vi "DHE_ReadTPs.vi"(5 "inRange":bool, 6 "index in":i32, 7 "value":string, 8 "error in (no error)":errorcluster, 9 "argument":string, 10 "action":T3=enum."GET ALL", 11 "file path":path=path "/home/arcconfig/TP_DHE.list") -> (0 "error out":errorcluster, 1 "index":i32[](array[numeric]), 2 "TPs":T1[](array[typedef]) {"Limits"."nominal" format="%.2f"; "Limits"."Lower" format="%.2f"; "Limits"."upper" format="%.2f"}, 3 "file path out":path=path "/home/ArcVIEW/ConfigFiles/PI_laboratory.cfg", 4 "devparams":string)   [LabVIEW 2016]
uses:
  DHE_TP_action.ctl
  DHE_TP.ctl
  DHE_TPLimits.ctl
  <vilib>/Utility/config.llb/Read Key (String).vi
  <vilib>/Utility/config.llb/NI_LVConfig.lvlib
panel:
  in  "DHE_TP":T1={"name"="", "type"="", "R_algor"=[], "board"="", "memory"="", "address"=0, "value"="", "Limits"={"upper"=9999999.0, "Lower"=-9999999.0, "InRange"=FALSE, "nominal"=0.0}, "unit"="", "params"="", "permissions"="RW", "W_algor"=[], "description"="", "err_count"=0, "max_err"=10, "read"=FALSE, "lowrej"=-9999999.0, "hirej"=9999999.0, "expupd"=FALSE} {"Limits"."nominal" format="%.2f"; "Limits"."Lower" format="%.2f"; "Limits"."upper" format="%.2f"}
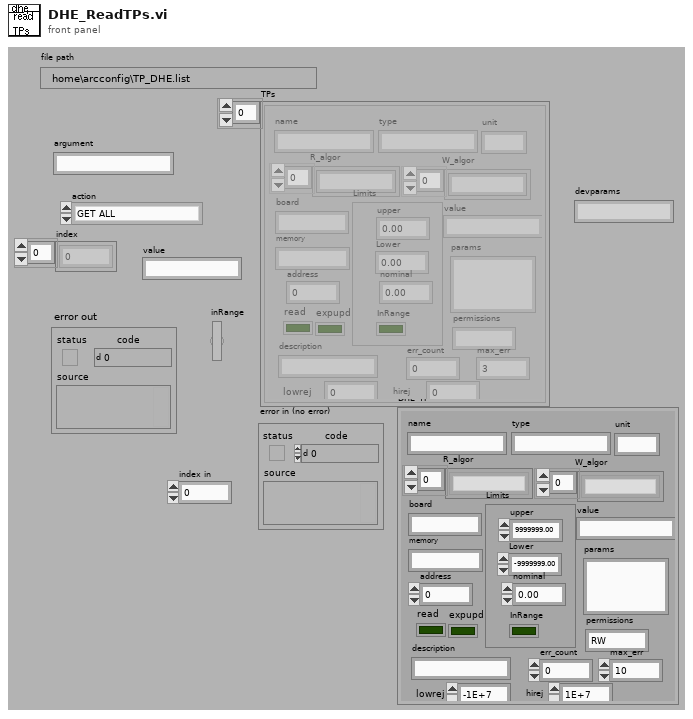
[diagram p1: front panel]
types:
  T1 = typedef "DHE_TP.ctl" = cluster{"name":string, "type":string, "R_algor":string[], "board":string, "memory":string, "address":i32, "value":string, "Limits":T2, "unit":string, "params":string, "permissions":string, "W_algor":string[], "description":string, "err_count":i32, "max_err":i32, "read":bool, "lowrej":dbl, "hirej":dbl, "expupd":bool}
  T2 = typedef "DHE_TPLimits.ctl" = cluster{"upper":dbl, "Lower":dbl, "InRange":bool, "nominal":dbl}
  T3 = typedef "DHE_TP_action.ctl" = enum16{"READ FROM FILE", "GET ALL", "FIND BY NAME", "FIND BY TYPE", "SET VALUE", "CLEAN", "CHANGE", "GET EXPUPDATE"}
  T4 = typedef "NI_LVConfig.lvlib/Config Data RefNum.ctl" = refnum<k1>
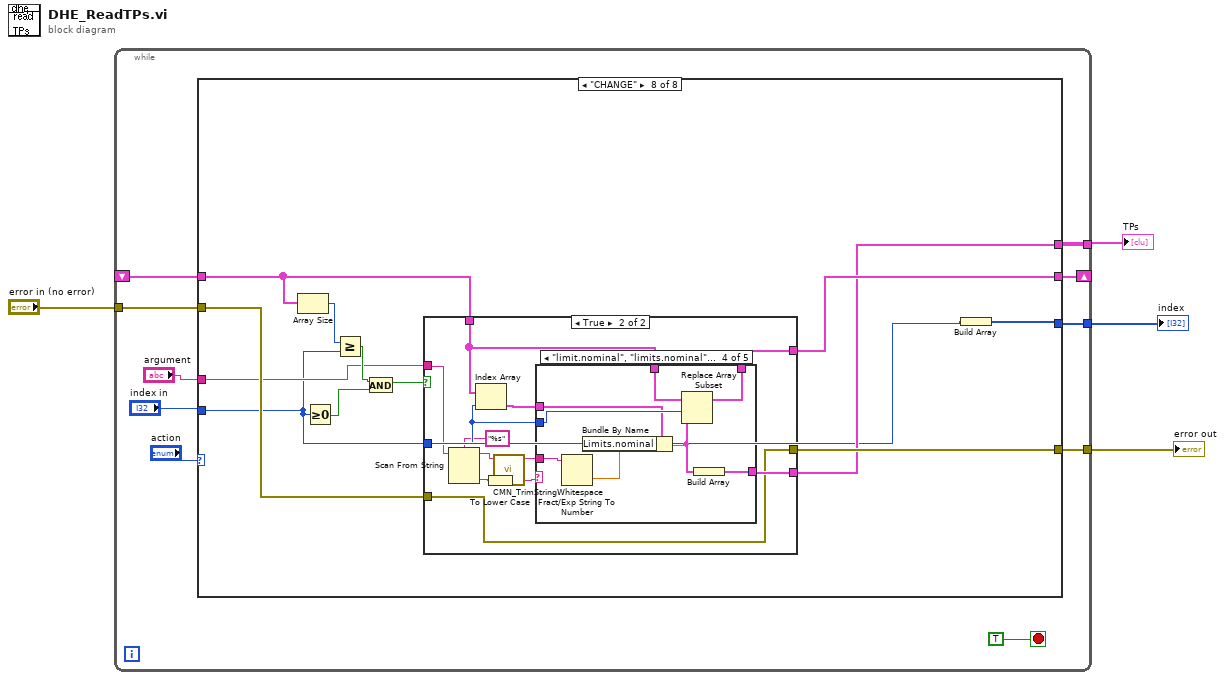
[diagram p0: block diagram]
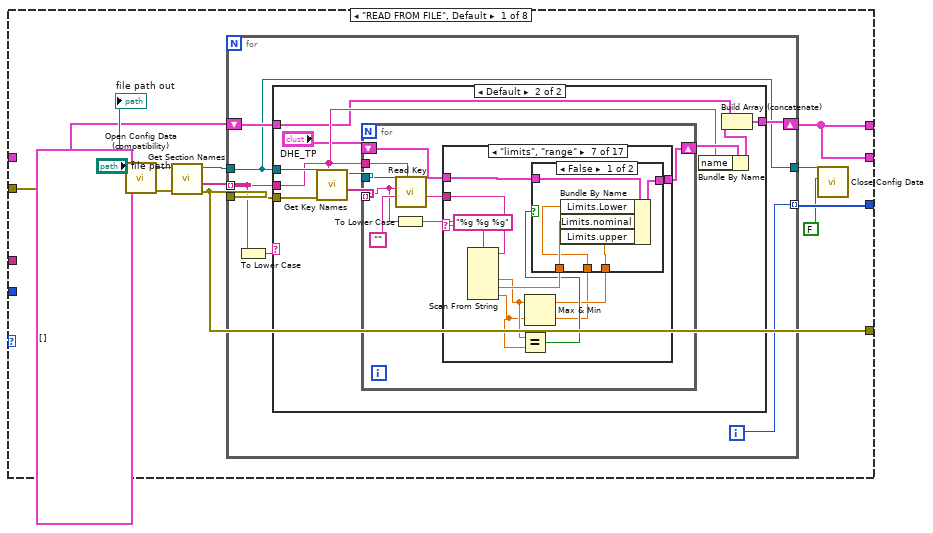
[diagram p2: hidden frame]
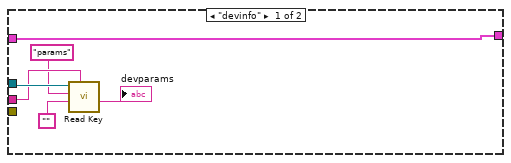
[diagram p3: hidden frame]
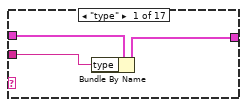
[diagram p4: hidden frame]
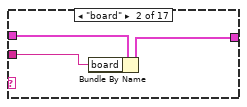
[diagram p5: hidden frame]
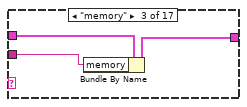
[diagram p6: hidden frame]
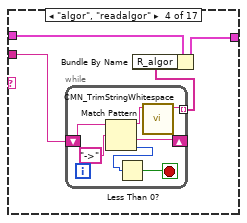
[diagram p7: hidden frame]
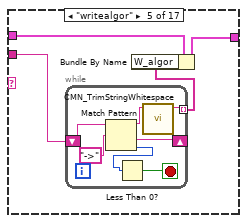
[diagram p8: hidden frame]
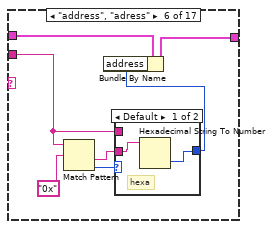
[diagram p9: hidden frame]
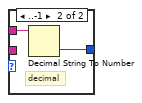
[diagram p10: hidden frame]
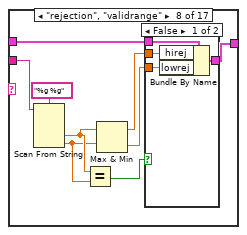
[diagram p12: hidden frame]
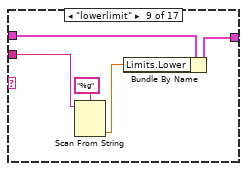
[diagram p14: hidden frame]
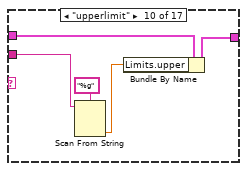
[diagram p15: hidden frame]
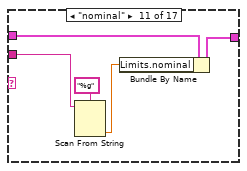
[diagram p16: hidden frame]
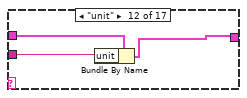
[diagram p17: hidden frame]
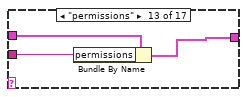
[diagram p18: hidden frame]
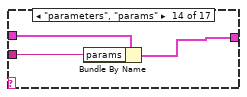
[diagram p19: hidden frame]
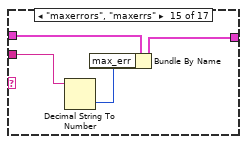
[diagram p20: hidden frame]
diagram:
  n1 = while {
    shift-right: [w11] -> _
    shift-left: _ -> [w10]
    tunnel: "error in (no error)" -> [w12]
    tunnel: [w8] -> w3
    tunnel: [w7] -> w2
    tunnel: [w6] -> w1
    stop <- TRUE stop-if-true
    n2 = case shown="\"CHANGE\"" "action" {
      tunnel: w12 -> [w25 w168 w175 w185 w190 w213 w261 w300]
      tunnel: [w18 w169 w174 w186 w193 w215 w263 w302] -> w11
      tunnel: w10 -> [_ w169 w174 _ w193 w215 w269 w308]
      tunnel: "argument" -> [_ _ _ _ w194 w216 _ w299]
      tunnel: [w20 w166 w170 i32[] [] w187 w211 w259 w297] -> w8
      tunnel: [w18 w169 w172 w186 w191 w214 w262 w301] -> w7
      tunnel: [w19 w168 w175 w185 w189 w212 w264 w303] -> w6
      tunnel: "index in" -> [_ _ _ _ _ _ w260 w298]
      frame "READ FROM FILE", Default {
        n3 = call <vilib>:"Open Config Data (compatibility).vi"("error in (no error)"=w25, "configuration file path"="file path") -> ("error out"=w24:errorcluster, "refnum"=w23:T4)  [unwired: 7 in, 1 out]
        n4 = call <vilib>:"Get Section Names.vi"("error in (no error)"=w24, "refnum"=w23) -> ("error out"=w19:errorcluster, "section names"=w21:string[], "refnum out"=w22:T4)  [unwired: 7 out]
        n5 = for {
          tunnel: w22 -> [w28]
          tunnel: w19 -> [w33]
          tunnel: w21 -> [w32] mode=indexing
          tunnel: [w27] -> w20 mode=indexing
          shift-right: [w30] -> w18
          shift-left: T1[] [] -> [w29]
          tunnel: [w28] -> w16
          i -> [w27]
          n6 = To Lower Case(string=w32) -> (all lower case string=w31:string)
          n7 = case shown="Default" w31 {
            tunnel: w28 -> [w38 w49]
            tunnel: w33 -> [_ w48]
            tunnel: w32 -> [w37 w44]
            tunnel: [w39 w41] -> w30
            tunnel: w29 -> [w39 w40]
            frame "devinfo" {
              n8 = call-poly <vilib>:"Read Key.vi"("section"=w37, "default value"="", "key"="params", "refnum"=w38) -> ("value"=→"devparams":string)  [unwired: 2 in, 5 out]
            }
            frame Default {
              n9 = call <vilib>:"Get Key Names.vi"("section"=w44, "error in (no error)"=w48, "refnum"=w49) -> ("key names"=w47:string[], "refnum out"=w46:T4)  [unwired: 7 out]
              n10 = for {
                tunnel: w47 -> [w53] mode=indexing
                tunnel: w44 -> [w56]
                tunnel: w46 -> [w55]
                shift-right: [w51] -> w45
                shift-left: "DHE_TP" -> [w50]
                n11 = To Lower Case(string=w53) -> (all lower case string=w57:string)
                n12 = call-poly <vilib>:"Read Key.vi"("section"=w56, "default value"="", "key"=w53, "refnum"=w55) -> ("value"=w52:string)  [unwired: 2 in, 5 out]
                n13 = case shown="\"limits\", \"range\"" w57 {
                  tunnel: w50 -> [w60 w63 w66 w70 w81 w95 w109 w119 w134 w139 w144 w147 w150 w153 w157 w162 w165]
                  tunnel: w52 -> [w59 w62 w65 w67 w78 w91 w107 w124 w132 w137 w142 w145 w148 w151 w155 w160 _]
                  tunnel: [w58 w61 w64 w69 w80 w94 w108 w118 w133 w138 w143 w146 w149 w152 w156 w161 w165] -> w51
                  frame "type" {
                    n14 = Bundle By Name(cluster=w60, "type"=w59) -> (w58:T1)
                  }
                  frame "board" {
                    n15 = Bundle By Name(cluster=w63, "board"=w62) -> (w61:T1)
                  }
                  frame "memory" {
                    n16 = Bundle By Name(cluster=w66, "memory"=w65) -> (w64:T1)
                  }
                  frame "algor", "readalgor" {
                    n17 = while {
                      tunnel: [w71] -> w68 mode=indexing
                      shift-right: [w74] -> _
                      shift-left: w67 -> [w73]
                      stop <- w75 stop-if-true
                      n18 = Match Pattern(string=w73, regular expression="->") -> (before substring=w72:string, after substring=w74:string, offset past match=w76:i32)  [unwired: 2 out]
                      n19 = Less Than 0?(x=w76) -> (x < 0?=w75:bool)
                      n20 = call "CMN_TrimStringWhitespace.vi"("string"=w72) -> ("trimmed string"=w71:string)  [unwired: 1 in, 8 out]
                    }
                    n21 = Bundle By Name(cluster=w70, "R_algor"=w68) -> (w69:T1)
                  }
                  frame "writealgor" {
                    n22 = while {
                      tunnel: [w82] -> w79 mode=indexing
                      shift-right: [w85] -> _
                      shift-left: w78 -> [w84]
                      stop <- w86 stop-if-true
                      n23 = Match Pattern(string=w84, regular expression="->") -> (before substring=w83:string, after substring=w85:string, offset past match=w87:i32)  [unwired: 2 out]
                      n24 = Less Than 0?(x=w87) -> (x < 0?=w86:bool)
                      n25 = call "CMN_TrimStringWhitespace.vi"("string"=w83) -> ("trimmed string"=w82:string)  [unwired: 1 in, 8 out]
                    }
                    n26 = Bundle By Name(cluster=w81, "W_algor"=w79) -> (w80:T1)
                  }
                  frame "address", "adress" {
                    n27 = Match Pattern(string=w91, regular expression="0x") -> (after substring=w89:string, offset past match=w92:i32)  [unwired: 3 out]
                    n28 = case shown="Default" w92 {
                      tunnel: w91 -> [_ w99]
                      tunnel: [w96 w98] -> w90
                      tunnel: w89 -> [w97 _]
                      frame Default {
                        # "hexa"
                        n29 = Hexadecimal String To Number(string=w97) -> (number=w96:u32)  [unwired: 3 out]
                      }
                      frame ..-1 {
                        # "decimal"
                        n30 = Decimal String To Number(string=w99) -> (number=w98:i32)  [unwired: 3 out]
                      }
                    }
                    n31 = Bundle By Name(cluster=w95, "address"=w90) -> (w94:T1)
                  }
                  frame "limits", "range" {
                    n32 = Scan From String(format string="%g %g %g", input string=w107) -> (output 1=w104:dbl, output 2=w105:dbl, output 3=w103:dbl)  [unwired: 2 in, 6 out]
                    n33 = Equal?(x=w104, y=w103) -> (x = y?=w102:bool)
                    n34 = Max & Min(x=w104, y=w103) -> (max(x,y)=w101:dbl, min(x,y)=w100:dbl)
                    n35 = case shown="False" w102 {
                      tunnel: w109 -> [w114 w115]
                      tunnel: [w113 w115] -> w108
                      tunnel: w105 -> [w112 _]
                      tunnel: w101 -> [w111 _]
                      tunnel: w100 -> [w110 _]
                      frame False {
                        n36 = Bundle By Name(cluster=w114, "Limits.Lower"=w110, "Limits.nominal"=w112, "Limits.upper"=w111) -> (w113:T1)
                      }
                      frame True {
                      }
                    }
                  }
                  frame "rejection", "validrange" {
                    n37 = Scan From String(format string="%g %g", input string=w124) -> (output 1=w122:dbl, output 2=w121:dbl)  [unwired: 2 in, 5 out]
                    n38 = Equal?(x=w122, y=w121) -> (x = y?=w120:bool)
                    n39 = Max & Min(x=w122, y=w121) -> (max(x,y)=w117:dbl, min(x,y)=w116:dbl)
                    n40 = case shown="False" w120 {
                      tunnel: w119 -> [w128 w129]
                      tunnel: [w127 w129] -> w118
                      tunnel: w117 -> [w126 _]
                      tunnel: w116 -> [w125 _]
                      frame False {
                        n41 = Bundle By Name(cluster=w128, "hirej"=w126, "lowrej"=w125) -> (w127:T1)
                      }
                      frame True {
                      }
                    }
                  }
                  frame "lowerlimit" {
                    n42 = Scan From String(format string="%g", input string=w132) -> (output 1=w130:dbl)  [unwired: 2 in, 4 out]
                    n43 = Bundle By Name(cluster=w134, "Limits.Lower"=w130) -> (w133:T1)
                  }
                  frame "upperlimit" {
                    n44 = Scan From String(format string="%g", input string=w137) -> (output 1=w135:dbl)  [unwired: 2 in, 4 out]
                    n45 = Bundle By Name(cluster=w139, "Limits.upper"=w135) -> (w138:T1)
                  }
                  frame "nominal" {
                    n46 = Scan From String(format string="%g", input string=w142) -> (output 1=w140:dbl)  [unwired: 2 in, 4 out]
                    n47 = Bundle By Name(cluster=w144, "Limits.nominal"=w140) -> (w143:T1)
                  }
                  frame "unit" {
                    n48 = Bundle By Name(cluster=w147, "unit"=w145) -> (w146:T1)
                  }
                  frame "permissions" {
                    n49 = Bundle By Name(cluster=w150, "permissions"=w148) -> (w149:T1)
                  }
                  frame "parameters", "params" {
                    n50 = Bundle By Name(cluster=w153, "params"=w151) -> (w152:T1)
                  }
                  frame "maxerrors", "maxerrs" {
                    n51 = Decimal String To Number(string=w155) -> (number=w154:i32)  [unwired: 3 out]
                    n52 = Bundle By Name(cluster=w157, "max_err"=w154) -> (w156:T1)
                  }
                  frame "expread", "expupdate" {
                    n53 = To Lower Case(string=w160) -> (all lower case string=w158:string)
                    n54 = case shown="\"1\", \"on\", \"true\", \"yes\"" w158 {
                      tunnel: [FALSE TRUE] -> w159
                      frame Default {
                      }
                      frame "1", "on", "true", "yes" {
                      }
                    }
                    n55 = Bundle By Name(cluster=w162, "expupd"=w159) -> (w161:T1)
                  }
                  frame Default {
                  }
                }
              }
              n56 = Bundle By Name(cluster=w45, "name"=w44) -> (w42:T1)
              n57 = Build Array (concatenate)(w40, w42) -> (w41:T1[])
            }
          }
        }
        n58 = call <vilib>:"Close Config Data.vi"("write file if changed (T)"=FALSE ("write configuration file? (T)"), "refnum"=w16) -> ()  [unwired: 1 in, 9 out]
        "file path out" <- "file path"
      }
      frame "GET ALL" {
        n59 = Array Size(array=w169) -> (size(s)=w167:i32)
        n60 = Build Array(w167) -> (w166:i32[])
      }
      frame "GET EXPUPDATE" {
        n61 = for {
          tunnel: w174 -> [w178] mode=indexing
          shift-right: [w177] -> w172
          shift-left: T1[] [] -> [w176]
          n62 = Unbundle By Name(w178) -> ("expupd"=w179:bool)
          n63 = case shown="False" w179 {
            tunnel: w178 -> [_ w183]
            tunnel: [w180 w182] -> w177
            tunnel: w176 -> [w180 w181]
            frame False {
            }
            frame True {
              n64 = Insert Into Array(array=w181, new element=w183) -> (w182:T1[])  [unwired: 1 in]
            }
          }
        }
        n65 = Array Size(array=w172) -> (size(s)=w171:i32)
        n66 = Build Array(w171) -> (w170:i32[])
      }
      frame "CLEAN" {
        w186 = T1[] []
      }
      frame "FIND BY NAME" {
        n67 = case shown="Default" w194 {
          tunnel: w193 -> [w207 _]
          tunnel: w194 -> [w206 _]
          tunnel: [w204 -1 ("f")] -> w192
          tunnel: [w205 T1[] [] ("tps")] -> w188
          tunnel: [w203 i32[] [] ("indexes")] -> w187
          frame Default {
            n68 = call "DHE_TP_parse_request.vi"("desired points"=w206, "TPs"=w207) -> ("indexes"=w203:i32[], "tps"=w205:T1[])  [unwired: 1 in, 7 out]
            n69 = Array Size(array=w203) -> (size(s)=w204:i32)
          }
          frame "", " " {
          }
        }
        n70 = case shown="Default" w192 {
          tunnel: [T1[] [] w201] -> w191
          tunnel: w190 -> [w197 w202]
          tunnel: [w196 w202] -> w189
          tunnel: w188 -> [_ w201]
          frame 0 {
            n71 = Bundle By Name(cluster=w197, "source"="TP NOT FOUND", "code"=-22, "status"=TRUE) -> (w196:errorcluster)
          }
          frame Default {
          }
        }
      }
      frame "FIND BY TYPE" {
        n72 = case shown="\"\", \" \"" w216 {
          tunnel: w215 -> [w226 _]
          tunnel: w216 -> [w225 _]
          tunnel: [w218 i32[] []] -> w211
          tunnel: [w223 T1[] []] -> w214
          tunnel: w213 -> [w221 w255]
          tunnel: [w220 w254] -> w212
          frame Default {
            n73 = for {
              tunnel: w226 -> [w238] mode=indexing
              tunnel: w225 -> [w243]
              shift-right: [w237] -> w223
              shift-left: T1[] [] -> [w236]
              shift-right: [w234] -> w218
              shift-left: i32[] [] -> [w233]
              i -> [w235]
              n74 = Unbundle By Name(w238) -> ("type"=w240:string)
              n75 = To Lower Case(string=w243) -> (all lower case string=w241:string)
              n76 = To Lower Case(string=w240) -> (all lower case string=w242:string)
              n77 = Equal?(x=w242, y=w241) -> (x = y?=w239:bool)
              n78 = case shown="True" w239 {
                tunnel: w238 -> [_ w251]
                tunnel: [w245 w250] -> w237
                tunnel: w236 -> [w245 w249]
                tunnel: w235 -> [_ w248]
                tunnel: [w244 w247] -> w234
                tunnel: w233 -> [w244 w246]
                frame False {
                }
                frame True {
                  n79 = Build Array (concatenate)(w249, w251) -> (w250:T1[])
                  n80 = Insert Into Array(array=w246, new element=w248) -> (w247:i32[])  [unwired: 1 in]
                }
              }
            }
            n81 = Array Size(array=w218) -> (size(s)=w217:i32)
            n82 = Greater Than 0?(x=w217) -> (x > 0?=w222:bool)
            n83 = case shown="False" w222 {
              tunnel: w221 -> [w231 w232]
              tunnel: [w227 w232] -> w220
              frame False {
                n84 = Bundle By Name(cluster=w231, "source"="TYPE NOT FOUND", "code"=-22, "status"=TRUE) -> (w227:errorcluster)
              }
              frame True {
              }
            }
          }
          frame "", " " {
            (unwired) T1 {"name"="", "type"="", "R_algor"=[], "board"="", "memory"="", "address"=0, "value"="", "Limits"={"upper"=0.0, "Lower"=0.0, "InRange"=FALSE, "nominal"=0.0}, "unit"="", "params"="", "permissions"="", "W_algor"=[], "description"="", "err_count"=0, "max_err"=0, "read"=FALSE, "lowrej"=0.0, "hirej"=0.0, "expupd"=FALSE} ("SDSU_TP")
            (unwired) -1 ("f")
            n85 = Bundle By Name(cluster=w255, "source"="TYPE NOT FOUND", "code"=-22, "status"=TRUE) -> (w254:errorcluster)
          }
        }
      }
      frame "SET VALUE" {
        n86 = Array Size(array=w269) -> (size(s)=w267:i32)
        n87 = Greater Or Equal To 0?(x=w260) -> (x >= 0?=w268:bool)
        n88 = Greater Or Equal?(x=w267, y=w260) -> (x >= y?=w266:bool)
        n89 = And(x=w266, y=w268) -> (x .and. y?=w265:bool)
        n90 = case shown="True" w265 {
          tunnel: w269 -> [w276 w295]
          tunnel: w260 -> [_ w293]
          tunnel: [w276 w294] -> w263
          tunnel: [w275 w285] -> w264
          tunnel: [T1[] [] w291] -> w262
          tunnel: w261 -> [w270 w285]
          frame False {
            n91 = Bundle By Name(cluster=w270, "status"=TRUE, "code"=-22, "source"="index out of range") -> (w275:errorcluster)
          }
          frame True {
            n92 = Index Array(array=w295, index=w293) -> (element=w284:T1)
            n93 = Scan From String(input string="value") -> (output 1=w277:dbl)  [unwired: 3 in, 4 out]
            n94 = Unbundle By Name(w284) -> ("hirej"=w280:dbl, "lowrej"=w279:dbl, "value"=w283:string)
            n95 = Unbundle By Name(w284) -> ("err_count"=w290:i32)
            n96 = Increment(x=w290) -> (x+1=w289:i32)
            n97 = In Range and Coerce(upper limit=w280, x=w277, lower limit=w279) -> (In Range?=w282:bool)  [unwired: 1 out]
            n98 = Select(t=w289, s=w285, f=0) -> (s? t:f=w288:i32)
            n99 = Select(t="value", s=w282, f=w283) -> (s? t:f=w281:string)
            n100 = Bundle By Name(cluster=w284, "read"=TRUE, "value"=w281, "Limits.InRange"="inRange", "err_count"=w288) -> (w292:T1)
            n101 = Replace Array Subset(array=w295, new element=w292, index=w293) -> (w294:T1[])
            n102 = Build Array(w292) -> (w291:T1[])
          }
        }
        n103 = Build Array(w260) -> (w259:i32[])
      }
      frame "CHANGE" {
        n104 = Array Size(array=w308) -> (size(s)=w306:i32)
        n105 = Greater Or Equal To 0?(x=w298) -> (x >= 0?=w307:bool)
        n106 = Greater Or Equal?(x=w306, y=w298) -> (x >= y?=w305:bool)
        n107 = And(x=w305, y=w307) -> (x .and. y?=w304:bool)
        n108 = case shown="True" w304 {
          tunnel: w308 -> [w315 w327]
          tunnel: w298 -> [_ w325]
          tunnel: [w315 w326] -> w302
          tunnel: [w314 w323] -> w303
          tunnel: [T1[] [] w324] -> w301
          tunnel: w300 -> [w309 w323]
          tunnel: w299 -> [_ w321]
          frame False {
            n109 = Bundle By Name(cluster=w309, "status"=TRUE, "code"=-22, "source"="index out of range") -> (w314:errorcluster)
          }
          frame True {
            n110 = Scan From String(format string="%s", input string=w321) -> (remaining string=w317:string, output 1=w319:string)  [unwired: 2 in, 3 out]
            n111 = Index Array(array=w327, index=w325) -> (element=w322:T1)
            n112 = To Lower Case(string=w319) -> (all lower case string=w318:string)
            n113 = call "CMN_TrimStringWhitespace.vi"("string"=w317) -> ("trimmed string"=w316:string)  [unwired: 1 in, 8 out]
            n114 = case shown="\"limit.nominal\", \"limits.nominal\", \"nominalvalue\"" w318 {
              tunnel: w327 -> [w329 w337 w345 w353 w361]
              tunnel: [w329 w336 w344 w352 w360] -> w326
              tunnel: w325 -> [_ w335 w343 w351 w359]
              tunnel: [T1[] [] w333 w341 w349 w357] -> w324
              tunnel: w322 -> [_ w332 w340 w348 w362]
              tunnel: w316 -> [_ w331 w339 w347 w364]
              frame Default {
              }
              frame "limit.lower", "limits.lower", "lowerlimit" {
                n115 = Fract/Exp String To Number(string=w331) -> (number=w330:dbl)  [unwired: 4 out]
                n116 = Bundle By Name(cluster=w332, "Limits.Lower"=w330) -> (w334:T1)
                n117 = Replace Array Subset(array=w337, new element=w334, index=w335) -> (w336:T1[])
                n118 = Build Array(w334) -> (w333:T1[])
              }
              frame "limit.upper", "limits.upper", "upperlimit" {
                n119 = Fract/Exp String To Number(string=w339) -> (number=w338:dbl)  [unwired: 4 out]
                n120 = Bundle By Name(cluster=w340, "Limits.upper"=w338) -> (w342:T1)
                n121 = Replace Array Subset(array=w345, new element=w342, index=w343) -> (w344:T1[])
                n122 = Build Array(w342) -> (w341:T1[])
              }
              frame "limit.nominal", "limits.nominal", "nominalvalue" {
                n123 = Fract/Exp String To Number(string=w347) -> (number=w346:dbl)  [unwired: 4 out]
                n124 = Bundle By Name(cluster=w348, "Limits.nominal"=w346) -> (w350:T1)
                n125 = Replace Array Subset(array=w353, new element=w350, index=w351) -> (w352:T1[])
                n126 = Build Array(w350) -> (w349:T1[])
              }
              frame "limits", "range" {
                n127 = Scan From String(format string="%g %g %g", input string=w364) -> (output 1=w356:dbl, output 2=w355:dbl, output 3=w354:dbl)  [unwired: 2 in, 6 out]
                n128 = Bundle By Name(cluster=w362, "Limits.Lower"=w356, "Limits.nominal"=w355, "Limits.upper"=w354) -> (w358:T1)
                n129 = Replace Array Subset(array=w361, new element=w358, index=w359) -> (w360:T1[])
                n130 = Build Array(w358) -> (w357:T1[])
              }
            }
          }
        }
        n131 = Build Array(w298) -> (w297:i32[])
      }
    }
  }
  "error out" <- w1
  "TPs" <- w2
  "index" <- w3
